vi "DS360 Set Frequency.vi"(8 "error in (no error)":T1, 10 "frequency":ext, 11 "GPIB address":string) -> (0 "error out":T1, 3 "address out":string)   [LabVIEW 2025, in "MyDS360.lvlib"]
uses:
  MyDS360.lvlib
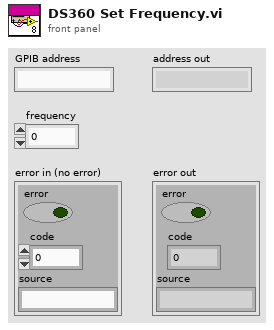
[diagram p1: front panel]
types:
  T1 = cluster{"error":bool, "code":i32, "source":string}
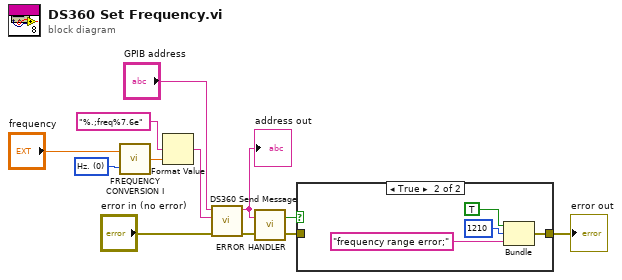
[diagram p0: block diagram]
diagram:
  w12 = 0 items=["Hz.", "KHz.", "MHz."] ("unit")
  n1 = call "FREQUENCY CONVERSION I.vi"("unit"=w12, "quantity"="frequency") -> ("output quantity"=w3:ext)
  n2 = Format Value(format string="%.;freq%7.6e", value (0)=w3) -> (output string=w4:string)  [unwired: 1 in]
  n3 = call "DS360 Send Message.vi"("address string"="GPIB address", "write buffer"=w4, "error in"="error in (no error)") -> ("address out"=w9:string, "error out"=w10:T1)  [unwired: 3 in, 2 out]
  "address out" <- w9
  n4 = call "ERROR HANDLER.vi"("error in"=w10, "GPIB address"=w9) -> ("error out"=w8:T1, "error found"=w7:bool)
  n5 = case shown="True" w7 {
    tunnel: w8 -> [w13 _]
    tunnel: [w13 w14] -> w11
    frame False {
    }
    frame True {
      n6 = Bundle(TRUE, 1210, "frequency range error;") -> (w14:errorcluster)  [unwired: 1 in]
    }
  }
  "error out" <- w11
